vi "start daemon.vi"(8 "error in (no error)":errorcluster) -> (0 "error out":errorcluster)   [LabVIEW 2020, in "ui-testing.lvlib"]
uses:
  ui-testing.lvlib
  main.vi
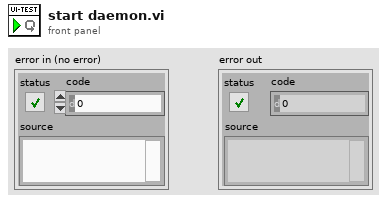
[diagram p1: front panel]
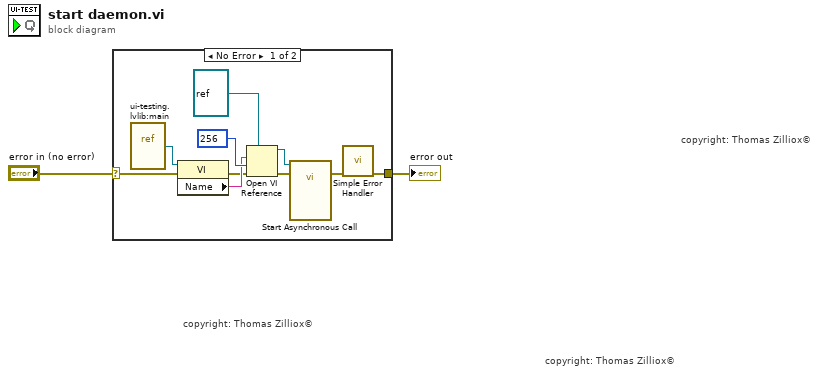
[diagram p0: block diagram]
diagram:
  # "copyright: Thomas Zilliox©"
  # "copyright: Thomas Zilliox©"
  # "copyright: Thomas Zilliox©"
  n1 = case shown="No Error" "error in (no error)" {
    selector: "error in (no error)" -> [w4 w13]
    tunnel: [w3 w13] -> w1
    frame No Error {
      n2 = vi-ref "ui-testing.lvlib:main.vi"() -> (w7:refnum<vi>)
      n3 = property class="VI"(reference=w7, error in=w4) -> (error out=w5:errorcluster, "Name"=w6:string)  [unwired: 1 out]
      n4 = Open VI Reference(type specifier VI Refnum (for type only)=refnum<vi> refnum, vi path=w6, options=256 ("call and forget"), error in (no error)=w5) -> (vi reference=w10:refnum<vi>, error out=w9:errorcluster)  [unwired: 2 in]
      n5 = call-by-ref "Start Asynchronous Call"(reference=w10, error in=w9) -> (error out=w8:errorcluster)  [unwired: 11 in, 2 out]
      n6 = call <vilib>:"Simple Error Handler.vi"("error in (no error)"=w8) -> ("error out"=w3:errorcluster)  [unwired: 4 in, 4 out]
    }
    frame Error {
    }
  }
  "error out" <- w1
